vi "KepcoDCPwr Configure List.vi"(0 "VISA Session":refnum<visa-resource-name>, 5 "Model In":string, 7 "channel name (\"\")":string="\"\"", 9 "List Type (DWell)":T1(ring)=enum."DWell List", 11 "error in (no error)":errorcluster {"code" format="%.0x"}, 12 "List":dbl[](array[numeric]) format="%^.6e") -> (4 "VISA Session Out":refnum<visa-resource-name>, 6 "Model Out":string, 8 "channel name out (\"\")":string="\"\"" caption="channel name Out (\"\")", 15 "error out":errorcluster {"code" format="%.0x"})   [LabVIEW 2013]
doc: "This VI configures the list.\n\nNote:\n\n1) This VI is available only for instruments with interface card BIT 4886."
uses:
  <vilib>/regexp/Match Regular Expression.xnode
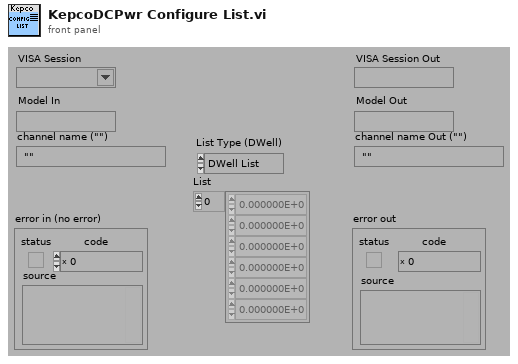
[diagram p1: front panel]
types:
  T1 = enum16{"Current List", "Voltage List", "DWell List"}
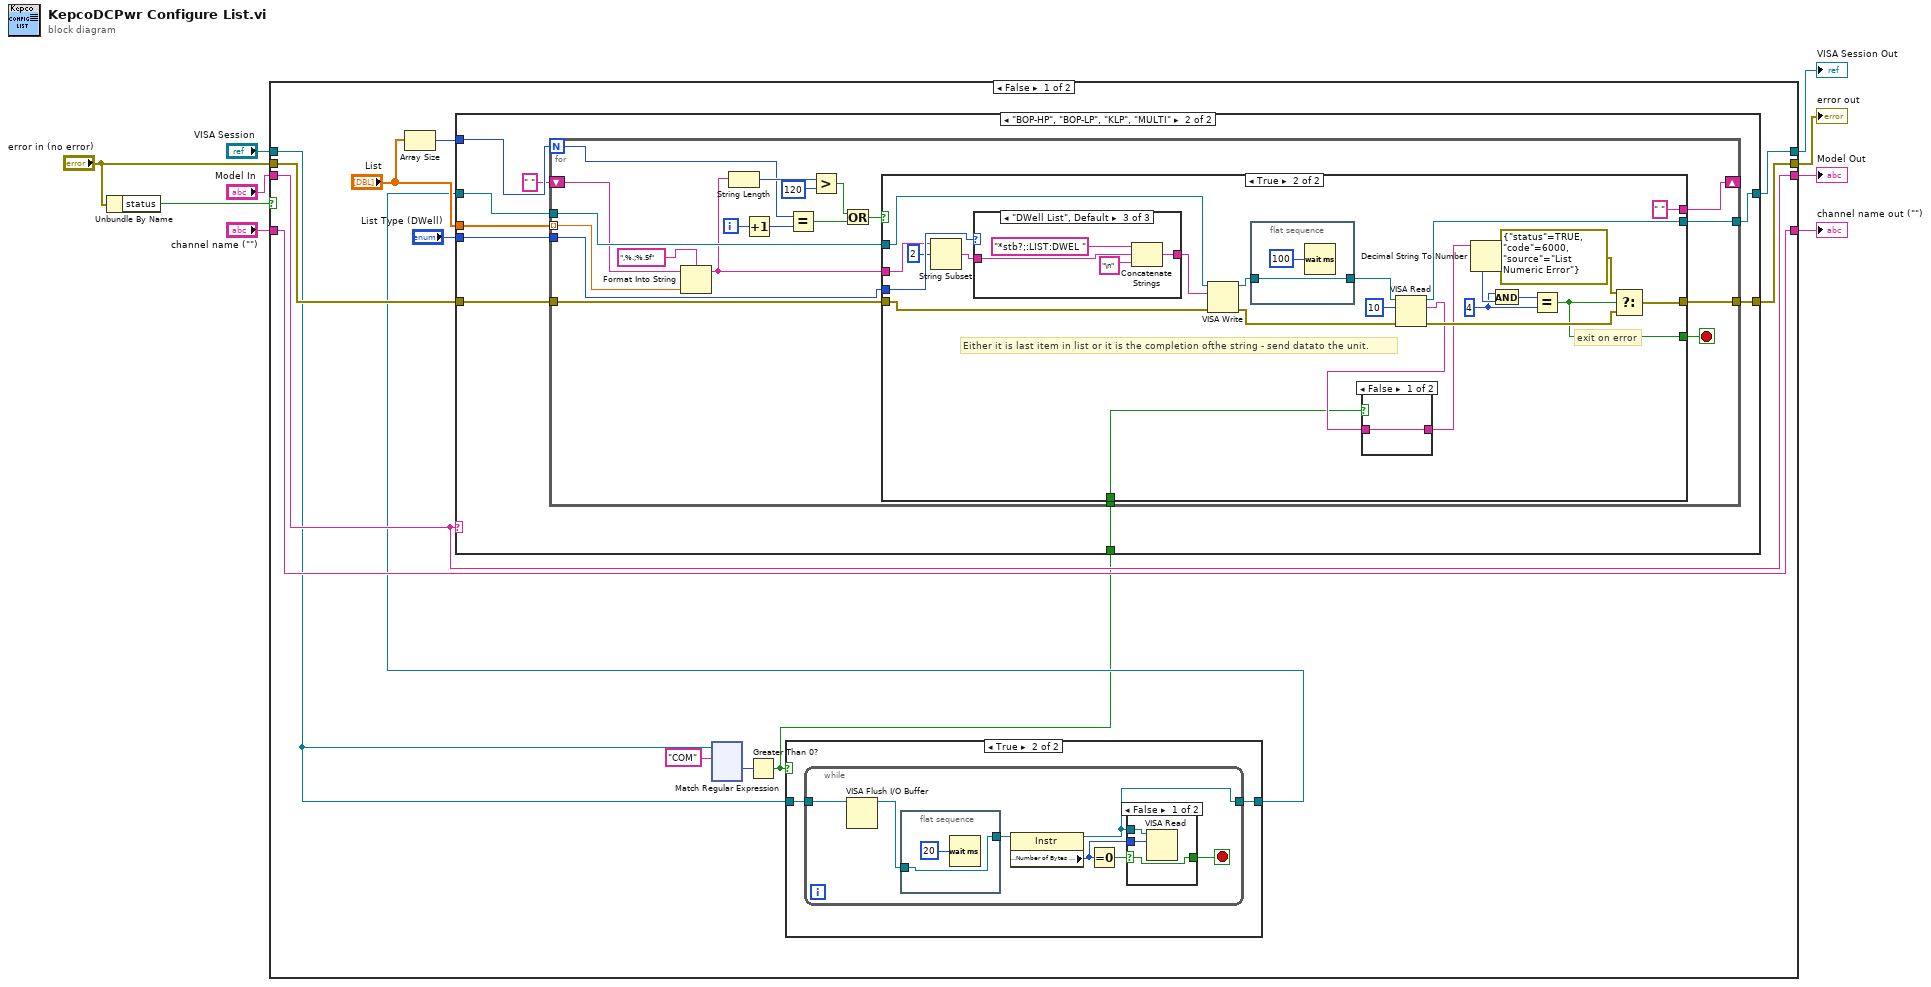
[diagram p0: block diagram]
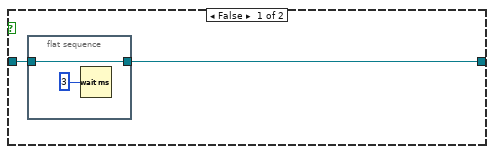
[diagram p2: hidden frame]
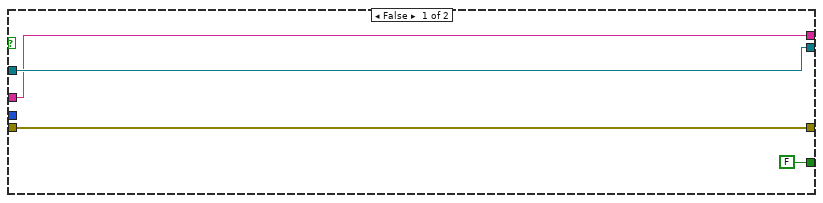
[diagram p5: hidden frame]
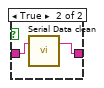
[diagram p6: hidden frame]
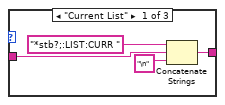
[diagram p7: hidden frame]
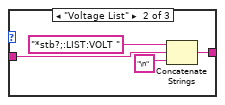
[diagram p8: hidden frame]
diagram:
  n1 = Unbundle By Name("error in (no error)") -> ("status"=w8:bool)
  n2 = case shown="False" w8 {
    tunnel: [w17 w230] -> w9
    tunnel: [w18 w231] -> w6
    tunnel: "VISA Session" -> [w11 w231]
    tunnel: "error in (no error)" -> [w20 w230]
    tunnel: [w21 w229] -> w3
    tunnel: "Model In" -> [w21 w229]
    tunnel: [w22 w228] -> w1
    tunnel: "channel name (\"\")" -> [w22 w228]
    frame False {
      n3 = Array Size(array="List") -> (size(s)=w15:i32)
      n4 = xnode "Match Regular Expression"("input string"=w11, "regular expression"="COM") -> ("offset past match"=w13:i32)  [unwired: 2 in, 6 out]
      n5 = Greater Than 0?(x=w13) -> (x > 0?=w10:bool)
      n6 = case shown="True" w10 {
        tunnel: [w24 w28] -> w12
        tunnel: w11 -> [w23 w27]
        frame False {
          n7 = flat-sequence {
            tunnel: w23 -> [w26]
            tunnel: [w26] -> w24
            frame #0 {
              n8 = Wait (ms)(milliseconds to wait=u32 3 ("byte count (0)")) -> ()  [unwired: 1 out]
            }
          }
        }
        frame True {
          n9 = while {
            tunnel: w27 -> [w31]
            tunnel: [w33] -> w28
            stop <- w34 stop-if-true
            n10 = VISA Flush I/O Buffer(VISA resource name=w31) -> (VISA resource name out=w30:refnum<visa-resource-name>)  [unwired: 2 in, 1 out]
            n11 = flat-sequence {
              tunnel: w30 -> [w36]
              tunnel: [w36] -> w29
              frame #0 {
                n12 = Wait (ms)(milliseconds to wait=u32 20) -> ()  [unwired: 1 out]
              }
            }
            n13 = property class="Instr"(reference=w29) -> (reference out=w33:refnum<visa-resource-name>, "Serial Settings:Number of Bytes at Serial Port"=w32:u32)  [unwired: 1 in, 1 out]
            n14 = Equal To 0?(x=w32) -> (x = 0?=w35:bool)
            n15 = case shown="False" w35 {
              selector: w35 -> [w40 w41]
              tunnel: [w40 w41] -> w34
              tunnel: w33 -> [w39 _]
              tunnel: w32 -> [w38 _]
              frame False {
                n16 = VISA Read(VISA resource name=w39, byte count=w38) -> ()  [unwired: 1 in, 4 out]
              }
              frame True {
              }
            }
          }
        }
      }
      n17 = case shown="\"BOP-HP\", \"BOP-LP\", \"KLP\", \"MULTI\"" w21 {
        tunnel: w20 -> [w154 w163]
        tunnel: w12 -> [w153 w162]
        tunnel: "List Type (DWell)" -> [_ w161]
        tunnel: "List" -> [_ w160]
        tunnel: [w153 w159] -> w18
        tunnel: [w154 w158] -> w17
        tunnel: w15 -> [_ w157]
        tunnel: w10 -> [_ w155]
        frame "", Default {
        }
        frame "BOP-HP", "BOP-LP", "KLP", "MULTI" {
          n18 = for {
            N: w157 -> [w172]
            tunnel: w163 -> [w183]
            tunnel: w162 -> [w182]
            tunnel: w161 -> [w181]
            tunnel: w160 -> [w168] mode=indexing
            tunnel: [w179] -> w159
            tunnel: [w180] -> w158
            shift-right: [w170] -> _
            shift-left: " " -> [w177]
            tunnel: w155 -> [w164]
            i -> [w166]
            stop <- w167 stop-if-true
            n19 = Format Into String(format string=",%.;%.5f", initial string=w177, w168) -> (resulting string=w169:string)  [unwired: 1 in, 1 out]
            n20 = String Length(string=w169) -> (length=w176:i32)
            n21 = Increment(x=w166) -> (x+1=w165:i32)
            n22 = Equal?(x=w172, y=w165) -> (x = y?=w173:bool)
            n23 = Greater?(x=w176, y=120) -> (0:w174:bool)
            n24 = Or(x=w174, y=w173) -> (x .or. y?=w171:bool)
            n25 = case shown="True" w171 {
              tunnel: w183 -> [w186 w210]
              tunnel: w182 -> [w187 w209]
              tunnel: w181 -> [_ w207]
              tunnel: [w186 w206] -> w180
              tunnel: [w187 w201] -> w179
              tunnel: [w184 " "] -> w170
              tunnel: w169 -> [w184 w194]
              tunnel: [FALSE w196] -> w167
              tunnel: w164 -> [_ w188]
              frame False {
              }
              frame True {
                w197 = u16 4 ("y")
                # "Either it is last item in list or it is the completion ofthe string - send datato the unit."
                # "exit on error"
                n26 = String Subset(string=w194, offset (0)=2) -> (substring=w193:string)  [unwired: 1 in]
                n27 = case shown="\"DWell List\", Default" w207 {
                  tunnel: [w217 w223 w226] -> w208
                  tunnel: w193 -> [w218 w221 w227]
                  frame "Current List" {
                    n28 = Concatenate Strings("*stb?;:LIST:CURR ", w218, "\n" ("string")) -> (w217:string)
                  }
                  frame "Voltage List" {
                    n29 = Concatenate Strings("*stb?;:LIST:VOLT ", w221, "\n" ("string")) -> (w223:string)
                  }
                  frame "DWell List", Default {
                    n30 = Concatenate Strings("*stb?;:LIST:DWEL ", w227, "\n" ("string")) -> (w226:string)
                  }
                }
                n31 = VISA Write(VISA resource name=w209, write buffer=w208, error in (no error)=w210) -> (VISA resource name out=w192:refnum<visa-resource-name>, error out=w203:errorcluster)  [unwired: 1 out]
                n32 = flat-sequence {
                  tunnel: [w214] -> w191
                  tunnel: w192 -> [w214]
                  frame #0 {
                    n33 = Wait (ms)(milliseconds to wait=u32 100) -> ()  [unwired: 1 out]
                  }
                }
                n34 = VISA Read(VISA resource name=w191, byte count=u32 10, error in (no error)=w203) -> (VISA resource name out=w201:refnum<visa-resource-name>, read buffer=w190:string, error out=w202:errorcluster)  [unwired: 1 out]
                n35 = case shown="False" w188 {
                  tunnel: w190 -> [w211 w212]
                  tunnel: [w211 w213] -> w189
                  frame False {
                  }
                  frame True {
                    n36 = call "Serial Data clean.vi"("string"=w212) -> ("Stripped of Xon Xoff"=w213:string)  [unwired: 2 in]
                  }
                }
                n37 = Decimal String To Number(string=w189) -> (number=w199:i32)  [unwired: 2 in, 1 out]
                n38 = And(x=w197, y=w199) -> (x .and. y?=w198:i32)
                n39 = Equal?(x=w198, y=w197) -> (x = y?=w196:bool)
                n40 = Select(t=errorcluster {"status"=TRUE, "code"=6000, "source"="List Numeric Error"}, s=w196, f=w202) -> (s? t:f=w206:errorcluster)
              }
            }
          }
        }
      }
    }
    frame True {
    }
  }
  "error out" <- w9
  "VISA Session Out" <- w6
  "channel name out (\"\")" <- w1
  "Model Out" <- w3
